vi "Shutter Operation (SubVI).vi"(0 "VISA resource name":refnum<visa-resource-name>, 1 "GPIO Pin":i32, 2 "Loop Iteration":i32, 3 "Delay (ms)":u32=20, 5 "error in (no error)":errorcluster, 6 "ON/OFF":bool, 8 "Manual Open":bool) -> (14 "VISA resource name out":refnum<visa-resource-name>, 19 "error out":errorcluster)   [LabVIEW 2018]
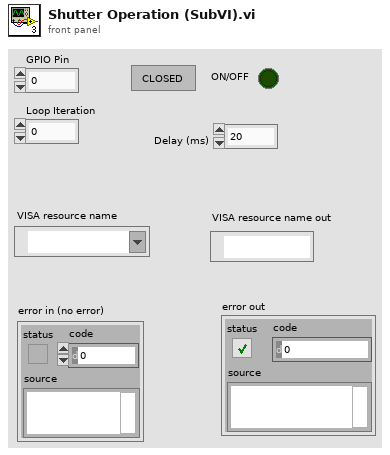
[diagram p1: front panel]
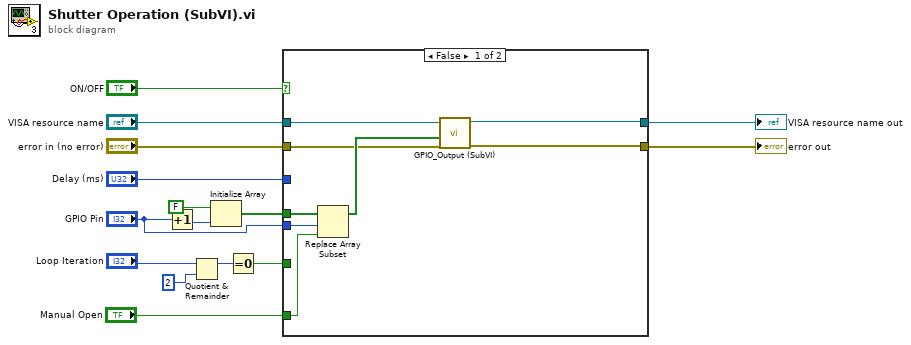
[diagram p0: block diagram]
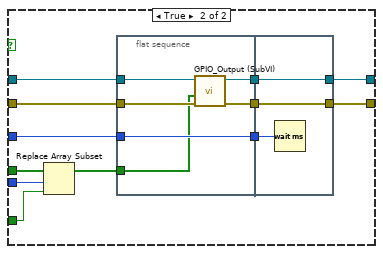
[diagram p2: hidden frame]
diagram:
  n1 = Increment(x="GPIO Pin") -> (x+1=w2:i32)
  n2 = Quotient & Remainder(x="Loop Iteration", y=2) -> (x-y*floor(x/y)=w14:i32)  [unwired: 1 out]
  n3 = Initialize Array(FALSE ("element"), w2) -> (w9:bool[])
  n4 = Equal To 0?(x=w14) -> (x = 0?=w5:bool)
  n5 = case shown="False" "ON/OFF" {
    tunnel: [w23 w33] -> w4
    tunnel: [w22 w32] -> w3
    tunnel: "Delay (ms)" -> [_ w30]
    tunnel: w9 -> [w21 w29]
    tunnel: "GPIO Pin" -> [w20 w28]
    tunnel: "VISA resource name" -> [w17 w27]
    tunnel: "error in (no error)" -> [w16 w26]
    tunnel: "Manual Open" -> [w18 _]
    tunnel: w5 -> [_ w25]
    frame False {
      n6 = Replace Array Subset(array=w21, new element=w18, index=w20) -> (w19:bool[])
      n7 = call "GPIO_Output (SubVI).vi"("error in (no error)"=w16, "GPIO Value"=w19, "VISA resource name"=w17) -> ("error out"=w22:errorcluster, "VISA resource name out"=w23:refnum<visa-resource-name>)  [unwired: 7 in]
    }
    frame True {
      n8 = Replace Array Subset(array=w29, new element=w25, index=w28) -> (w24:bool[])
      n9 = flat-sequence {
        tunnel: [w41] -> w35
        tunnel: [w40] -> w34
        tunnel: w30 -> [w39]
        tunnel: [w39] -> w31
        tunnel: w27 -> [w38]
        tunnel: w26 -> [w37]
        tunnel: w24 -> [w36]
        tunnel: [w44] -> w33
        tunnel: w35 -> [w44]
        tunnel: [w43] -> w32
        tunnel: w34 -> [w43]
        tunnel: w31 -> [w42]
        frame #0 {
          n10 = call "GPIO_Output (SubVI).vi"("error in (no error)"=w37, "GPIO Value"=w36, "VISA resource name"=w38) -> ("error out"=w40:errorcluster, "VISA resource name out"=w41:refnum<visa-resource-name>)  [unwired: 7 in]
        }
        frame #1 {
          n11 = Wait (ms)(milliseconds to wait=w42) -> ()  [unwired: 1 out]
        }
      }
    }
  }
  "VISA resource name out" <- w4
  "error out" <- w3
